vi "2_Power_Transmission_Line_Fault_Classification(Inference).vi"() -> ()   [LabVIEW 2020]
uses:
  <vilib>/Ngene/DeepLTK/Toolkit/NN_Network/Controls/NN_Save_Before_Destroy_Options.ctl
  <vilib>/Ngene/DeepLTK/Toolkit/NN_Layers/Layers/Input/API/NN_Layer_Set_Out(Input1D_idx).vi
  <vilib>/Ngene/DeepLTK/Toolkit/Deep_Learning_Toolkit_by_Ngene.lvlib
  <vilib>/measure/NI_MABase.lvlib
panel:
  in  "Position":sgl(slide)=0.49211356 scale=0.0..1.0
  in  "Fault Generation":T1(tab)=enum."Transient"
  in  "scale":sgl(slide)=0.5 scale=0.5..0.65
  in  "Duration(#s)":i32(slide)=600 scale=300.0..600.0
  in  "scale":sgl(slide)=1.50625 scale=1.4..1.6
  in  "Duration(#s)":i32(slide)=415 scale=300.0..600.0
  in  "Duration(#s)":i32(slide)=400 scale=200.0..600.0
  in  "Tau":sgl(slide)=150.0 scale=130.0..150.0
  in  "Frequency":sgl(slide)=2000.0 scale=500.0..1500.0
  in  "Amplitude":sgl(slide)=137.5 scale=100.0..150.0
  in  "Offset":sgl(slide)=107.291664 scale=50.0..150.0
  in  "Duration(#s)":i32(slide)=385 scale=200.0..600.0
  out "Predicted Class":string="Transient"
  out "Class Labels":string[](array[string])=["DC Offset", "Interruption", "Normal", "Sag", "Swell", "Transient"]
  out "Generated WaveForm":waveform(sgl)(graph)={"t0"=timestamp(0 s since 1904-01-01), "dt"=1.0, "Y"=array[2000 elements]}
  in  "Weight File Path":path=path "D:/Ngene/GitHub/deepltk_examples/2_Waveform_Processing/23_Power_Transmission_Line_Fault_Classification/working/Fault_Classifier/Fault_Classifier_weights_23_11_07__17_39_46.bin"
  in  "Configuration File Path":path=path "D:/Ngene/GitHub/deepltk_examples/2_Waveform_Processing/23_Power_Transmission_Line_Fault_Classification/working/Fault_Classifier/Fault_Classifier_net_cfg_23_11_07__17_39_46.cfg"
  out "Class Probabilities":sgl[](array[slide])=[8.41936e-24, 0.0, 0.00047341821, 7.864271e-11, 1.1491938e-11, 0.9995266] scale=0.0..1.0
  in  "Stop":bool
  # "Overview: Demonstrates the usage of DeepLTK for loading the model pretrained for Power Line Fault Classification and running for inference.\nRequirements: DeepLTK - Deep Learning Toolkit for LabVIEW (https://www.ngene.co/deep-learning-toolkit-for-labview)\nInstructions:\n1. Provide Network Configuration File Path and Weight File Path generated from training example.\n2. Run the VI\n3. Choose type of the fault and change the parameters and observe the predicted type of the fault.\n4. Press the Stop button to stop the VI.\n\nMore Examples:  https://github.com/ngenehub/deepltk_examples"
  # "Power Transmission Line Fault Classification - Inference"
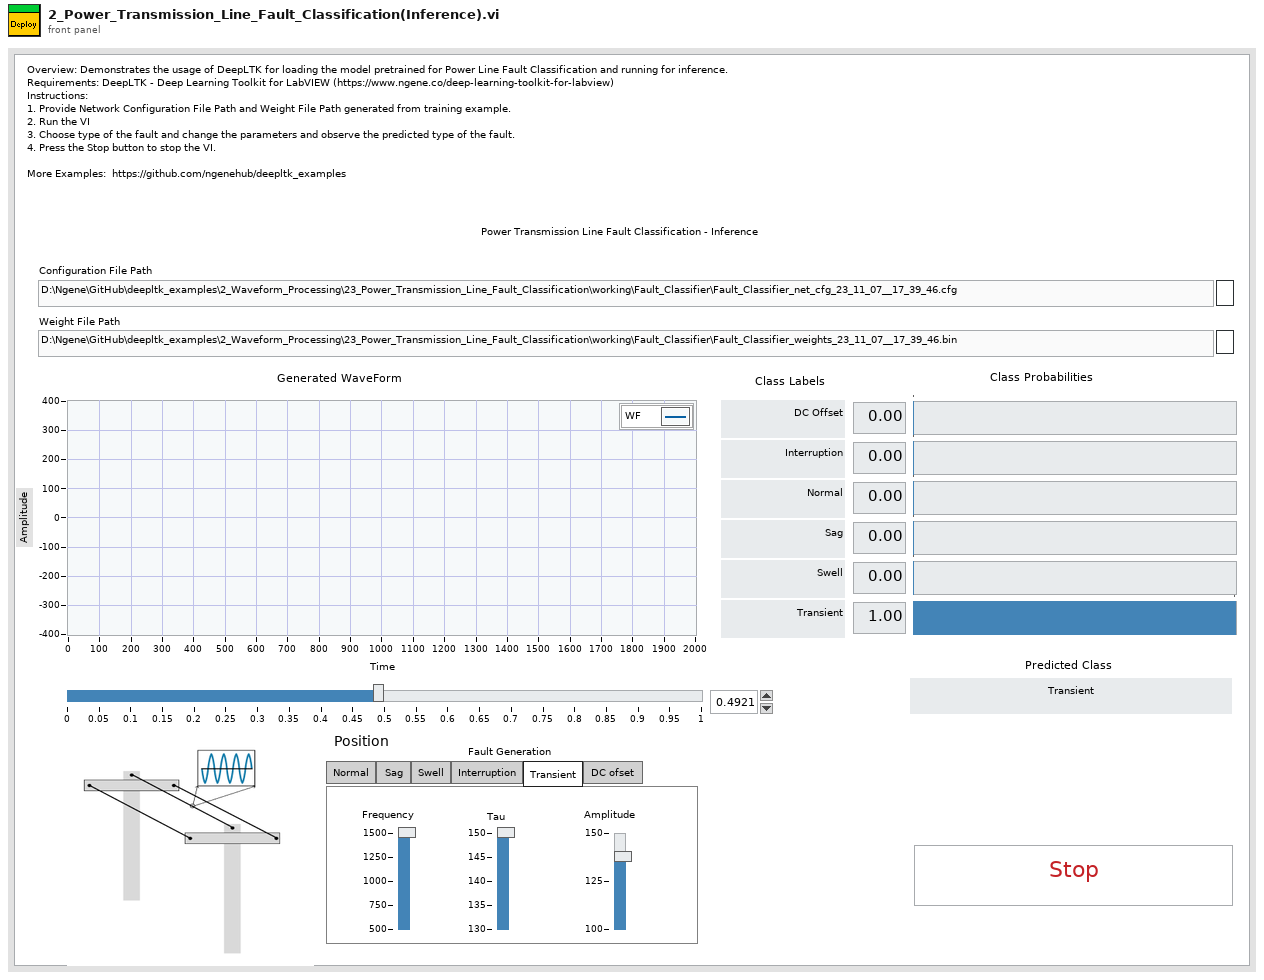
[diagram p1: front panel]
types:
  T1 = enum32{"Normal", "Sag ", "Swell", "Interruption", "Transient", "DC ofset "}
  T2 = typedef "Deep_Learning_Toolkit_by_Ngene.lvlib/NN_Save_Before_Destroy_Options.ctl" = cluster{"CFG?":bool, "Weights?":bool, "Render?":bool}
  T3 = typedef "Deep_Learning_Toolkit_by_Ngene.lvlib/NN_Config_Params.ctl" = cluster{"Name":string, "mBatch":i32, "NN_Train_Params":T4, "LR_Decay_Policy":T7, "Labels":string[], "Loss":T9}
  T4 = typedef "Deep_Learning_Toolkit_by_Ngene.lvlib/NN_Train_Params.ctl" = cluster{"Optimizer":T5, "Beta_1":sgl, "Beta_2":sgl, "Weight Decay(L1)":sgl, "Weight Decay(L2)":sgl, "Data_Sampling":T6}
  T5 = typedef "Deep_Learning_Toolkit_by_Ngene.lvlib/NN_Train_Optimizer.ctl" = enum16{"SGD", "Adam", "Adagrad", "Adadelta", "RMSProp", "Nesterov"}
  T6 = typedef "Deep_Learning_Toolkit_by_Ngene.lvlib/NN_Train_Data_Sampling.ctl" = enum16{"Random", "Sequential"}
  T7 = typedef "Deep_Learning_Toolkit_by_Ngene.lvlib/NN_LR_Policy_Cfg.ctl" = cluster{"Policy_Type":T8, "LR0":dbl, "k":sgl, "WarmUp_Policy":enum16{"Step", "Ramp"}, "WarmUp_Iter":i32, "WarmUp_Ratio":sgl}
  T8 = typedef "Deep_Learning_Toolkit_by_Ngene.lvlib/NN_LR_Policy_Type.ctl" = enum16{"Manual", "Step", "Exp", "1/t"}
  T9 = typedef "Deep_Learning_Toolkit_by_Ngene.lvlib/NN_Loss_Config_Params.ctl" = cluster{"Loss_Type":T10, "Loss_Conf_Params":variant}
  T10 = typedef "Deep_Learning_Toolkit_by_Ngene.lvlib/NN_Loss_Type.ctl" = enum16{"None", "MSE", "CrossEntropy", "YOLO_v2"}
  T11 = typedef "Deep_Learning_Toolkit_by_Ngene.lvlib/NN_Layer_Config_Params.ctl" = cluster{"Layer_Type":T12, "Layer_Conf_Params":variant}
  T12 = typedef "Deep_Learning_Toolkit_by_Ngene.lvlib/NN_Layer_Type.ctl" = enum16{"Input1D", "Input3D", "Conv2D", "Conv2D_Adv", "MaxPool", "AvgPool", "UpSample", "DropOut3D", "ShortCut", "Concat", "SoftMax3D", "FC", "DropOut", "Softmax", "Flatten", "YOLO_v2", "Unsupported"}
  T13 = typedef "Deep_Learning_Toolkit_by_Ngene.lvlib/NN.ctl" = cluster{"Name":string, "No of Layers":i32, "mBatch":i32, "Layers":T14[], "Dimty":T15, "Dims_In":T16, "Dims_Out":T16, "Working_Dir":path, "Train?":bool, "Train_Params":T4, "LR_Update_Policy":T7, "Session Data":T17, "Ground_truth":T18, "NNg_hdls":T20, "NN_Device":T21, "GPU Id":i32, "Labels":string[], "Receptive Field":T22[], "Loss_Type":T10, "Loss_Cfg_Prms":variant}
  T14 = typedef "Deep_Learning_Toolkit_by_Ngene.lvlib/NN_Layer_ref.ctl" = refnum<data-value>
  T15 = typedef "Deep_Learning_Toolkit_by_Ngene.lvlib/NN_In_Out_Dim-ty.ctl" = enum8{"In1D_Out1D", "In3D_Out1D", "In3D_Out3D", "In3D_OutBBox"}
  T16 = typedef "Deep_Learning_Toolkit_by_Ngene.lvlib/NN_Dims(C,H,W).ctl" = cluster{"C":i32, "H":i32, "W":i32}
  T17 = typedef "Deep_Learning_Toolkit_by_Ngene.lvlib/NN_Train_Session_Data.ctl" = cluster{"Epochs":sgl, "Tot_Iter":i32, "LR":sgl, "LR_iter":i32}
  T18 = typedef "Deep_Learning_Toolkit_by_Ngene.lvlib/NN_Ground_truth.ctl" = cluster{"Y":variant, "Y_idx":T19}
  T19 = typedef "Deep_Learning_Toolkit_by_Ngene.lvlib/NN_Data_ref(1D_I32).ctl" = refnum<data-value>
  T20 = typedef "Deep_Learning_Toolkit_by_Ngene.lvlib/nng_cuda_handles.ctl" = cluster{"cudnn":u64, "cublas":u64, "stream":u64, "curand":u64}
  T21 = typedef "Deep_Learning_Toolkit_by_Ngene.lvlib/NN_Device.ctl" = enum16{"CPU", "GPU"}
  T22 = typedef "Deep_Learning_Toolkit_by_Ngene.lvlib/NN_Dims(V,H).ctl" = cluster{"V":i32, "H":i32}
  T23 = typedef "Deep_Learning_Toolkit_by_Ngene.lvlib/NN_Layer.ctl" = cluster{"Name":string, "Layer_Data":variant, "Layer_Type":T12, "Dims_In":T16, "Layers_In":variant, "Dims_Out":T16, "Layers_Out":variant, "Metrics":T24, "GPU_Data":variant, "mBatch":i32, "NN_Device":T21, "NNg_hdls":T20, "Train?":bool, "Dimty":T25, "RecptField":T26}
  T24 = typedef "Deep_Learning_Toolkit_by_Ngene.lvlib/NN_Layer_Metrics.ctl" = cluster{"Data":dbl, "Params":dbl, "Ops":dbl}
  T25 = typedef "Deep_Learning_Toolkit_by_Ngene.lvlib/NN_Layer_Dimty.ctl" = enum16{"1D", "3D"}
  T26 = typedef "Deep_Learning_Toolkit_by_Ngene.lvlib/NN_Layer_RF_State.ctl" = cluster{"Dims":T22, "J":T22}
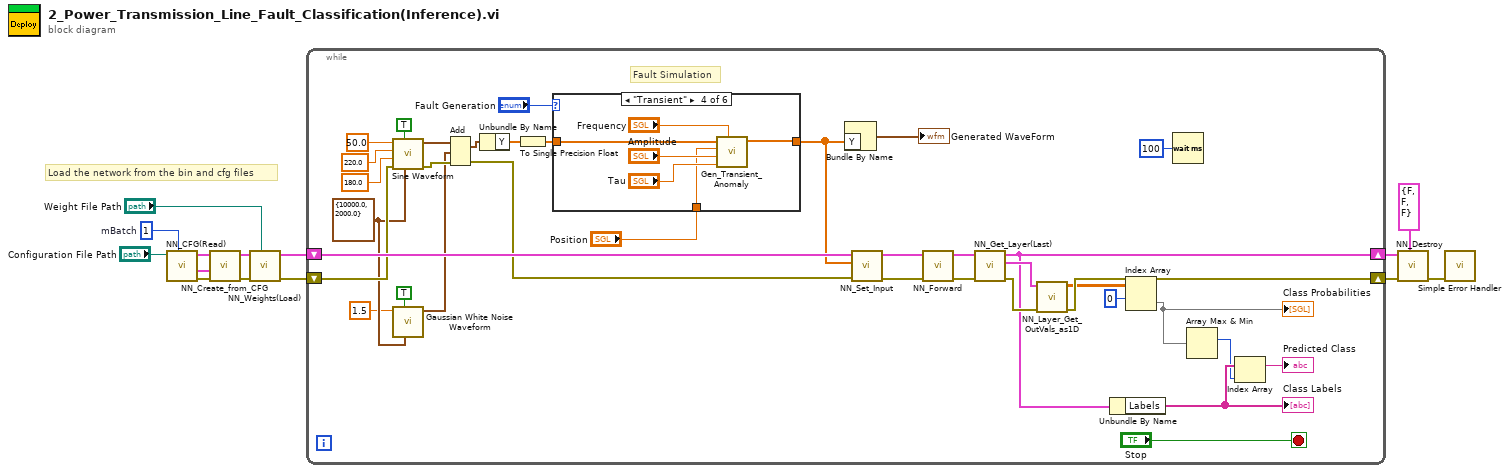
[diagram p0: block diagram]
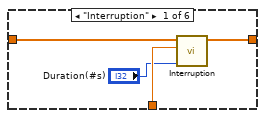
[diagram p2: hidden frame]
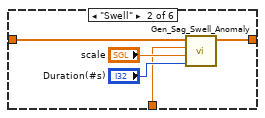
[diagram p3: hidden frame]
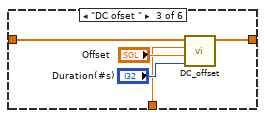
[diagram p4: hidden frame]
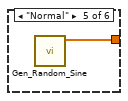
[diagram p5: hidden frame]
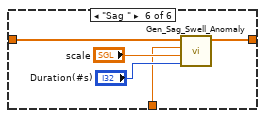
[diagram p6: hidden frame]
diagram:
  w1 = 1  # mBatch
  # "Load the network from the bin and cfg files"
  n1 = call <vilib>:"NN_CFG(Read).vi"("mBatch"=w1, "CFG file path"="Configuration File Path") -> ("error out"=w8:errorcluster, "Net_Cfg"=w9:T3, "Layer_Cfg"=w7:T11[])  [unwired: 7 in]
  n2 = call <vilib>:"NN_Create_from_CFG.vi"("error in (no error)"=w8, "Net_Cfg"=w9, "Layer_Cfg"=w7) -> ("error out"=w11:errorcluster, "NN out"=w6:T13)  [unwired: 7 in]
  n3 = call <vilib>:"NN_Weights(Load).vi"("Weight File Path"="Weight File Path", "error in (no error)"=w11, "NN in"=w6) -> ("error out"=w5:errorcluster, "NN out"=w4:T13)  [unwired: 7 in]
  n4 = while {
    shift-right: [w50] -> w14
    shift-left: w5 -> [w23]
    shift-right: [w39] -> w13
    shift-left: w4 -> [w40]
    stop <- "Stop" stop-if-true
    w21 = cluster{"Fs":dbl, "#s":dbl} {"Fs"=10000.0, "#s"=2000.0} ("sampling info")
    # "Fault Simulation"
    n5 = call <vilib>:"Sine Waveform.vi"("sampling info"=w21, "reset signal"=TRUE, "error in (no error)"=w23, "phase"=180.0, "amplitude"=220.0, "frequency"=50.0) -> ("error out"=w17:errorcluster, "signal out"=w32:waveform(dbl))  [unwired: 4 in]
    n6 = call <vilib>:"Gaussian White Noise Waveform.vi"("sampling info"=w21, "reset signal"=TRUE, "standard deviation"=sgl 1.5 ("Noise Standart Deviation")) -> ("signal out"=w15:waveform(dbl))  [unwired: 7 in, 1 out]
    n7 = Add(1:w15, 2:w32, 4:w17) -> (0:w19:waveform(dbl), 3:w16:errorcluster)
    n8 = Unbundle By Name(w19) -> ("Y"=w31:dbl[])
    n9 = To Single Precision Float(number=w31) -> (single precision float=w27:sgl[])
    n10 = case shown="\"Transient\"" "Fault Generation" {
      tunnel: [w53 w56 w61 w69 w71 w73] -> w29
      tunnel: w27 -> [w54 w59 w64 w70 _ w76]
      tunnel: "Position" -> [w52 w55 w60 w65 _ w72]
      frame "Interruption" {
        n11 = call "Interruption.vi"("Duration"="Duration(#s)", "Position"=w52, "Sine"=w54) -> ("Sine+Anomaly"=w53:sgl[])  [unwired: 8 in]
      }
      frame "Swell" {
        n12 = call "Gen_Sag_Swell_Anomaly.vi"("Duration"="Duration(#s)", "Amplitude"="scale", "Position"=w55, "Sine"=w59) -> ("Sine+Anomaly"=w56:sgl[])  [unwired: 7 in]
      }
      frame "DC ofset " {
        n13 = call "DC_offset.vi"("Duration"="Duration(#s)", "Ampltude"="Offset", "Position"=w60, "Sine"=w64) -> ("Sine+Anomaly"=w61:sgl[])  [unwired: 7 in]
      }
      frame "Transient" {
        n14 = call "Gen_Transient_Anomaly.vi"("Frequency"="Frequency", "Tau"="Tau", "Amplitude"="Amplitude", "Position"=w65, "Sine"=w70) -> ("Sine+Anomaly"=w69:sgl[])  [unwired: 6 in]
      }
      frame "Normal" {
        n15 = call "Gen_Random_Sine.vi"() -> ("data"=w71:sgl[])  [unwired: 11 in]
      }
      frame "Sag " {
        n16 = call "Gen_Sag_Swell_Anomaly.vi"("Duration"="Duration(#s)", "Amplitude"="scale", "Position"=w72, "Sine"=w76) -> ("Sine+Anomaly"=w73:sgl[])  [unwired: 7 in]
      }
    }
    n17 = Bundle By Name("Y"=w29) -> (→"Generated WaveForm":waveform(sgl))  [unwired: 1 in]
    n18 = call-poly <vilib>:"NN_Set_Input.vi"("error in (no error)"=w16, "Data_In(1D_SGL)"=w29, "NN In"=w40) -> ("error out"=w49:errorcluster, "NN Out"=w46:T13)  [unwired: 7 in]
    n19 = call <vilib>:"NN_Forward.vi"("error in (no error)"=w49, "NN in"=w46) -> ("error out"=w48:errorcluster, "NN out"=w47:T13)  [unwired: 6 in, 2 out]
    n20 = call <vilib>:"NN_Get_Layer(Last).vi"("error in (no error)"=w48, "NN in"=w47) -> ("error out"=w45:errorcluster, "Last_Layer"=w44:T23, "NN out"=w39:T13)  [unwired: 6 in, 1 out]
    n21 = call <vilib>:"NN_Layer_Get_OutVals_as1D.vi"("error in (no error)"=w45, "Layer"=w44) -> ("error out"=w50:errorcluster, "Out(as1D)"=w43:sgl[][])  [unwired: 8 in]
    n22 = Unbundle By Name(w39) -> ("Labels"=w36:string[])
    "Class Labels" <- w36
    n23 = Index Array(array=w43, index (row)=0) -> (element=w37:sgl[])  [unwired: 1 in]
    "Class Probabilities" <- w37
    n24 = Wait (ms)(milliseconds to wait=u32 100) -> ()  [unwired: 1 out]
    n25 = Array Max & Min(array=w37) -> (max index (indices)=w35:i32)  [unwired: 3 out]
    n26 = Index Array(array=w36, index=w35) -> (element=→"Predicted Class":string)
  }
  n27 = call <vilib>:"NN_Destroy.vi"("Save (T, T, T)"=T2 {"CFG?"=FALSE, "Weights?"=FALSE, "Render?"=FALSE}, "error in (no error)"=w14, "NN in"=w13) -> ("error out"=w2:errorcluster)  [unwired: 8 in]
  n28 = call <vilib>:"Simple Error Handler.vi"("error in (no error)"=w2) -> ()  [unwired: 4 in, 5 out]
